vi "52_RC Servo Motor_adj.vi"() -> ()   [LabVIEW 2018]
uses:
  <userlib>/KNR OS 4.0 LabVIEW Toolkit/Type Definition/Resource.ctl
  <userlib>/KNR OS 4.0 LabVIEW Toolkit/Type Definition/RC Servo Port.ctl
panel:
  in  "IP":string(combo)="172.22.11.2"
  in  "RC Motor":T1=3 items=["RC_onboard"=3, "RC_box"=9]
  in  "Resource":T2=enum."KNRm_DDDD"
  in  "stop":bool
  in  "RC Pulse Width (uS)":u16[](array[slide])=[1500, 1500, 1500, 1500, 1500, 1500, 1500] scale=500.0..2500.0
  # "700~2300"
  # "295~2652"
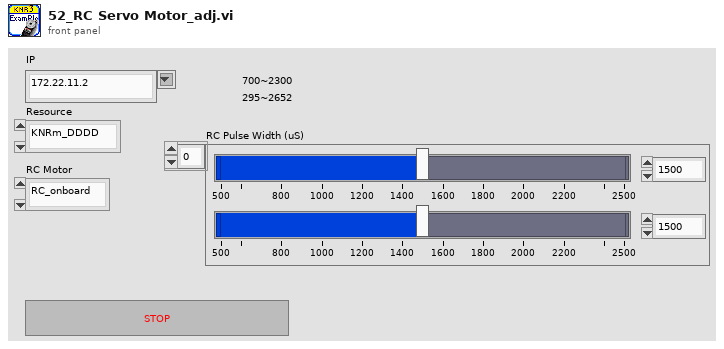
[diagram p1: front panel]
types:
  T1 = typedef "RC Servo Port.ctl" = u16
  T2 = typedef "Resource.ctl" = enum16{"KNRm_DDRC", "KNRm_DDDD", "KNRm_DDDR", "KNRm_DDDC", "KNR", "KNRm_neww"}
  T3 = typedef "KNR3 Reference.ctl" = cluster{"FPGA Session":refnum<class "FPGA Interface Base.lvclass">, "Resource":T2}
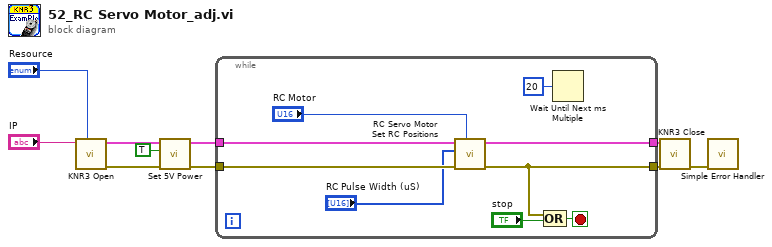
[diagram p0: block diagram]
diagram:
  n1 = call <userlib>:"KNR3 Open.vi"("Resource"="Resource", "IP"="IP") -> ("error out"=w7:errorcluster, "KNR out"=w10:T3)  [unwired: 8 in]
  n2 = call <userlib>:"Set 5V Power.vi"("error in (no error)"=w7, "5V Power(T)"=TRUE ("5V Power"), "KNR in"=w10) -> ("error out"=w6:errorcluster, "KNR out"=w9:T3)  [unwired: 7 in]
  n3 = while {
    tunnel: w9 -> [w19]
    tunnel: [w18] -> w8
    tunnel: w6 -> [w17]
    tunnel: [w13] -> w5
    stop <- w15 stop-if-true
    n4 = call <userlib>:"RC Servo Motor Set RC Positions.vi"("Port (RC_onboard)"="RC Motor", "error in (no error)"=w17, "RC Pulse Width (1500 uS)"="RC Pulse Width (uS)", "KNR in"=w19) -> ("error out"=w13:errorcluster, "KNR out"=w18:T3)  [unwired: 6 in]
    n5 = Compound Arithmetic op=OR(w13, "stop") -> (w15:bool)
    n6 = Wait Until Next ms Multiple(millisecond multiple=u32 20) -> ()  [unwired: 1 out]
  }
  n7 = call <userlib>:"KNR3 Close.vi"("error in (no error)"=w5, "KNR in"=w8) -> ("error out"=w4:errorcluster)  [unwired: 9 in]
  n8 = call <vilib>:"Simple Error Handler.vi"("error in (no error)"=w4) -> ()  [unwired: 4 in, 5 out]
